vi "Street Illumination Problem.vi"() -> ()   [LabVIEW 2023]
doc: "Determines the illumination power of two street lights at a particular point on the street."
uses:
  <vilib>/gmath/NI_Gmath.lvlib
panel:
  in  "Stop":bool
  in  "Tab Control":enum32{"Example", "Theory"}(tab)
  in  "P1[W]":dbl=2000.0
  in  "P2[W]":dbl=3000.0
  in  "h1[m]":dbl=5.0
  in  "h2[m]":dbl=6.0
  in  "s[m]":dbl=20.0
  out "Illumination Intensity":cluster{"X Values":dbl[], "Y Values":dbl[]}[](graph)
  out "C1(x)=C2(x)":dbl format="%#.6g"
  out "f(C1(x)=C2(x))":dbl format="%#.6g"
  out "Minimum":dbl format="%#.6g"
  out "f(Minimum)":dbl format="%#.6g"
  in  "Formulas":string[](array[string])=["(P1*H1)/sqrt((H1^2+x^2))^3", "(P2*H2)/sqrt((H2^2+(S-x)^2))^3"]
  # "Overview: Determines how to perform calculations pertaining to the illumination power of two street lights at a particular point on the street with various 1D & 2D Evaluation VIs.\nRequirements: LabVIEW Full Development System\nInstructions: \n1. Run the VI.\n2. Observe the Illumination Intensity graph. Switch to the Theory tab for more information about the formulas used for the calculations.\n3. Click Stop to stop the VI."
  # "Illumination Problem"
  # "A road is illuminated by two lights, where P1 denotes the illumination power and h1 the height of the first light, P2 and h2 of the second light.\n\nThe total illumination at point x can be calculated by:"
  # "Figure out the x with minimal illumination. Here, s is the distance between the two lights."
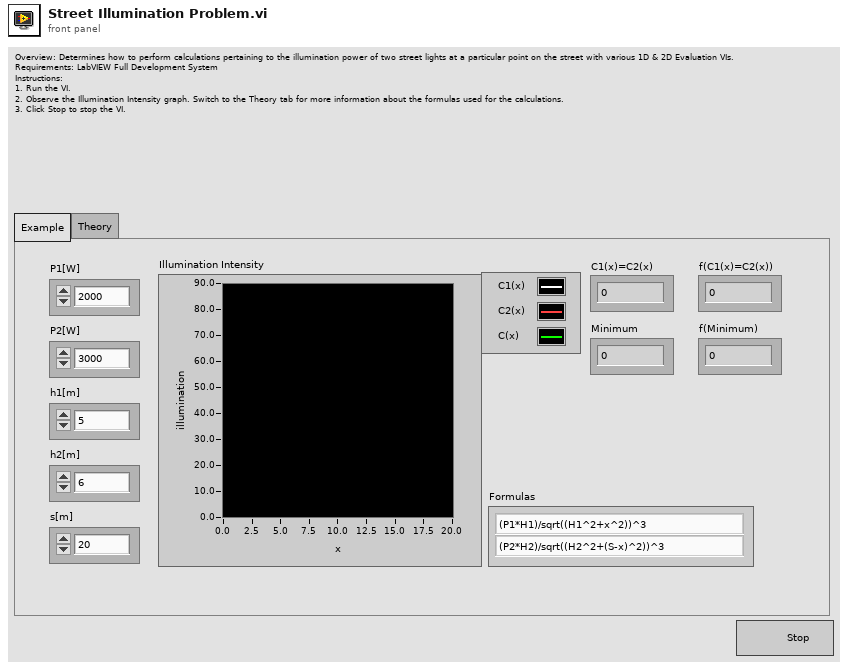
[diagram p1: front panel]
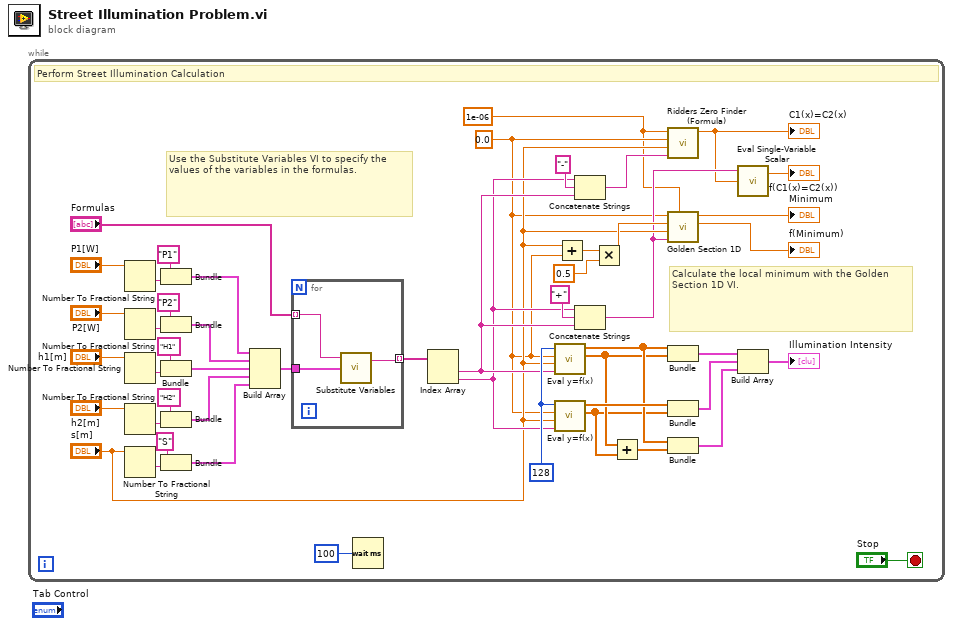
[diagram p0: block diagram]
diagram:
  n1 = while {
    stop <- "Stop" stop-if-true
    w3 = 1e-06
    w4 = 0.0
    w49 = u32 128 ("# of points")
    # "Calculate the local minimum with the Golden Section 1D VI."
    # "Use the Substitute Variables VI to specify the values of the variables in the formulas."
    # "Perform Street Illumination Calculation"
    n2 = Number To Fractional String(number="P1[W]") -> (F-format string=w29:string)  [unwired: 3 in]
    n3 = Number To Fractional String(number="P2[W]") -> (F-format string=w26:string)  [unwired: 3 in]
    n4 = Number To Fractional String(number="h1[m]") -> (F-format string=w22:string)  [unwired: 3 in]
    n5 = Number To Fractional String(number="h2[m]") -> (F-format string=w25:string)  [unwired: 3 in]
    n6 = Number To Fractional String(number="s[m]") -> (F-format string=w20:string)  [unwired: 3 in]
    n7 = Bundle("P1", w29) -> (w16:cluster{string, string})  [unwired: 1 in]
    n8 = Bundle("P2", w26) -> (w15:cluster{string, string})  [unwired: 1 in]
    n9 = Bundle("H1", w22) -> (w14:cluster{string, string})  [unwired: 1 in]
    n10 = Bundle("H2", w25) -> (w13:cluster{string, string})  [unwired: 1 in]
    n11 = Bundle("S", w20) -> (w12:cluster{string, string})  [unwired: 1 in]
    n12 = Build Array(w16, w15, w14, w13, w12) -> (w11:cluster{string, string}[])
    n13 = for {
      tunnel: "Formulas" -> [w53] mode=indexing
      tunnel: w11 -> [w51]
      tunnel: [w52] -> w48 mode=indexing
      n14 = call <vilib>:"Substitute Variables.vi"("Substitution Rules"=w51, "original formula"=w53) -> ("formula after substitution"=w52:string)  [unwired: 1 in, 1 out]
    }
    n15 = Wait (ms)(milliseconds to wait=u32 100) -> ()  [unwired: 1 out]
    n16 = Index Array(array=w48) -> (element #1=w37:string, element #2=w9:string)  [unwired: 2 in]
    n17 = call <vilib>:"Eval y=f(x).vi"("formula"=w37, "end"="s[m]", "start"=w4, "number of points"=w49) -> ("Y Values"=w45:dbl[], "X Values"=w46:dbl[])  [unwired: 2 out]
    n18 = call <vilib>:"Eval y=f(x).vi"("formula"=w9, "end"="s[m]", "start"=w4, "number of points"=w49) -> ("Y Values"=w44:dbl[], "X Values"=w47:dbl[])  [unwired: 2 out]
    n19 = Add(x="s[m]", y=w4) -> (x+y=w35:dbl)
    n20 = Concatenate Strings(w9, "-", w37) -> (w31:string)
    n21 = Concatenate Strings(w9, "+", w37) -> (w7:string)
    n22 = Multiply(x=w35, y=0.5) -> (x*y=w34:dbl)
    n23 = Add(x=w45, y=w44) -> (x+y=w43:dbl[])
    n24 = call <vilib>:"Ridders Zero Finder (Formula).vi"("formula"=w31, "end"="s[m]", "start"=w4, "accuracy"=w3) -> ("zero"=w6:dbl)  [unwired: 4 in, 3 out]
    "C1(x)=C2(x)" <- w6
    n25 = call <vilib>:"Golden Section 1D.vi"("accuracy"=w3, "formula"=w7, "c (start)"="s[m]", "b (start)"=w34, "a (start)"=w4) -> ("f(minimum)"=→"f(Minimum)":dbl, "minimum"=→"Minimum":dbl)  [unwired: 2 out]
    n26 = Bundle("X Values"=w46, "Y Values"=w45) -> (w42:cluster{"X Values":dbl[], "Y Values":dbl[]})  [unwired: 1 in]
    n27 = Bundle("X Values"=w47, "Y Values"=w44) -> (w41:cluster{"X Values":dbl[], "Y Values":dbl[]})  [unwired: 1 in]
    n28 = Bundle("X Values"=w46, w43) -> (w40:cluster{"X Values":dbl[], dbl[]})  [unwired: 1 in]
    n29 = call <vilib>:"Eval Single-Variable Scalar.vi"("x value"=w6, "formula"=w7) -> ("y value"=→"f(C1(x)=C2(x))":dbl)  [unwired: 1 in, 1 out]
    n30 = Build Array(w42, w41, w40) -> (→"Illumination Intensity":cluster{"X Values":dbl[], "Y Values":dbl[]}[])
  }
